vi "To File (Path).vi"(6 "Pretty Print?":bool=TRUE, 7 "enable LabVIEW extensions? (T)":bool=TRUE, 8 "error in (no error)":errorcluster, 10 "JSON Value in":variant, 11 "path in":path) -> (0 "error out":errorcluster, 3 "path out":path)   [LabVIEW 2017, in "Advanced Variant Tools.lvlib"]
doc: "Saves a JSON instance's data to the given file."
uses:
  Advanced Variant Tools.lvlib
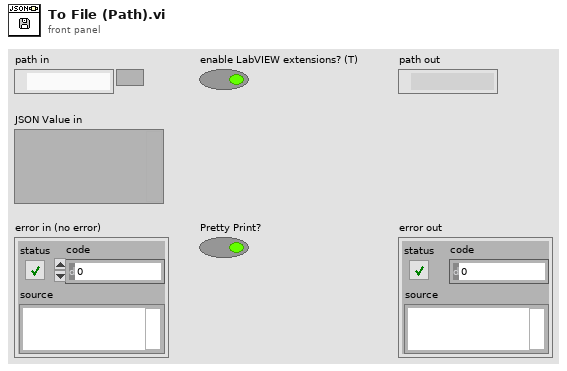
[diagram p1: front panel]
types:
  T1 = enum16{"open", "replace", "create", "open or create", "replace or create", "replace or create with confirmation"}
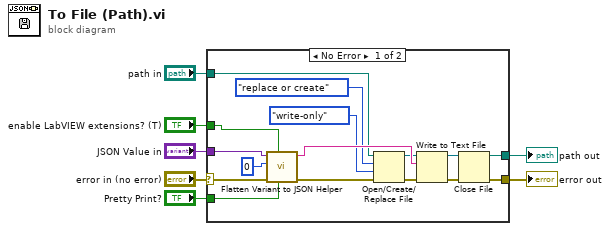
[diagram p0: block diagram]
diagram:
  n1 = case shown="No Error" "error in (no error)" {
    selector: "error in (no error)" -> [w18 w25]
    tunnel: "JSON Value in" -> [w23 _]
    tunnel: "path in" -> [w16 w24]
    tunnel: [w15 w25] -> w4
    tunnel: "Pretty Print?" -> [w12 _]
    tunnel: "enable LabVIEW extensions? (T)" -> [w13 _]
    tunnel: [w9 w24] -> w1
    frame No Error {
      n2 = call "Flatten Variant to JSON Helper.vi"("pretty print? (T)"=w12, "enable LabVIEW extensions? (T)"=w13, "error in (no error)"=w18, "indent"=0, "JSON Value in"=w23) -> ("error out"=w14:errorcluster, "String"=w22:string)  [unwired: 5 in]
      n3 = Open/Create/Replace File(file path (use dialog)=w16, error in=w14, operation (0:open)=T1."replace or create", access (0:read/write)=enum16{"read/write", "read-only", "write-only"}."write-only") -> (refnum out=w19:refnum<file>, error out=w17:errorcluster)  [unwired: 2 in, 1 out]
      n4 = Write to Text File(file (use dialog)=w19, text=w22, error in=w17) -> (refnum out=w20:refnum<file>, error out=w21:errorcluster)  [unwired: 1 in, 1 out]
      n5 = Close File(refnum=w20, error in=w21) -> (path=w9:path, error out=w15:errorcluster)
    }
    frame Error {
    }
  }
  "error out" <- w4
  "path out" <- w1
